vi "MNK_Z_Bridge_to_DSC.vi"(8 "error in (no error)":errorcluster, 9 "calibration string":string, 10 "description string":string, 11 "dbl":dbl[](array[numeric])) -> (0 "error out":errorcluster)   [LabVIEW 2016]
panel:
  in  "calibration string var":refnum<k21>="ni.var.psp://housesoftheholy/MNK_18T/MNK_TC_Z_calibration"
  in  "description string var":refnum<k21>="ni.var.psp://housesoftheholy/MNK_18T/MNK_TC_Z_description"
  in  "dbl var":refnum<k21>[](array[refnum])=["ni.var.psp://housesoftheholy/MNK_18T/MNK_Cstill_Z", "ni.var.psp://housesoftheholy/MNK_18T/MNK_CMN-187_Z", "ni.var.psp://housesoftheholy/MNK_18T/MNK_Cstill_T", "ni.var.psp://housesoftheholy/MNK_18T/MNK_CMN-187_T"]
  # "MNK Impedence Bridge to DSC"
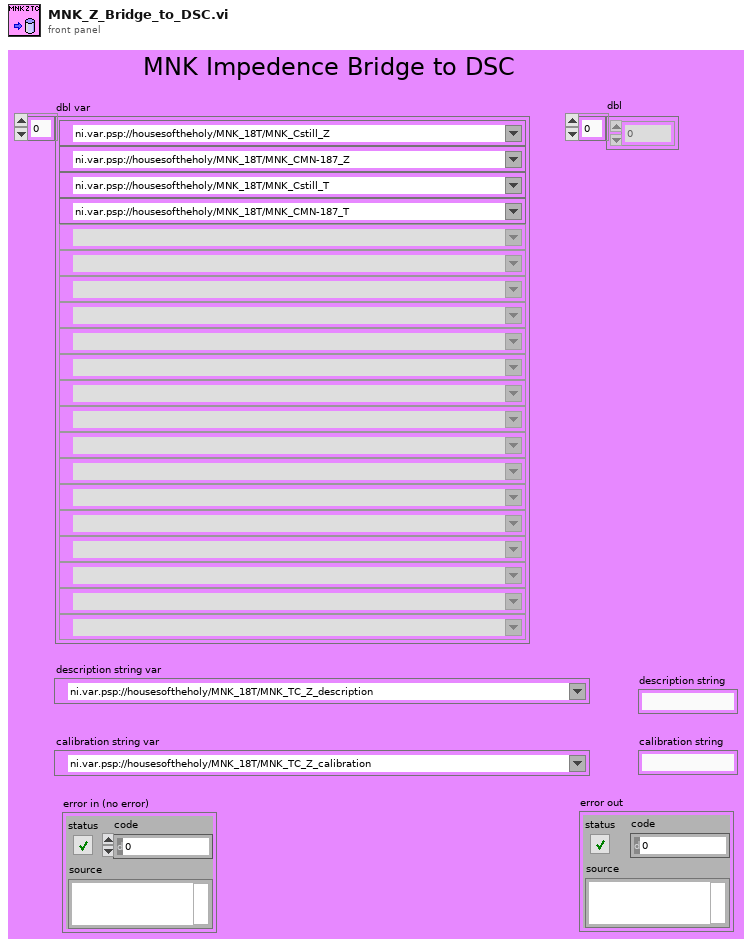
[diagram p1: front panel]
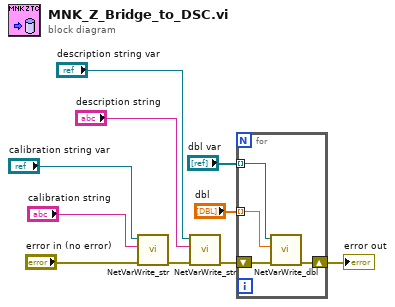
[diagram p0: block diagram]
diagram:
  n1 = call "NetVarWrite_str.vi"("error in (no error)"="error in (no error)", "String"="calibration string", "Refnum in"="calibration string var") -> ("error out"=w1:errorcluster)  [unwired: 8 in]
  n2 = call "NetVarWrite_str.vi"("error in (no error)"=w1, "String"="description string", "Refnum in"="description string var") -> ("error out"=w5:errorcluster)  [unwired: 8 in]
  n3 = for {
    tunnel: "dbl var" -> [w14] mode=indexing
    tunnel: "dbl" -> [w13] mode=indexing
    shift-right: [w11] -> w8
    shift-left: w5 -> [w12]
    n4 = call "NetVarWrite_dbl.vi"("error in (no error)"=w12, "Numeric"=w13, "Refnum in"=w14) -> ("error out"=w11:errorcluster)  [unwired: 8 in]
  }
  "error out" <- w8
